vi "Main Page.vi"(8 "error in (no error)":errorcluster, 11 "Node Ptr":T3 format="%.0x") -> (0 "error out":errorcluster)   [LabVIEW 2026, in "Nominal Core Streaming System Explorer.lvlib"]
uses:
  Nominal Core Streaming System Explorer.lvlib
  <vilib>/NI VeriStand/Custom Device API/Custom Device Item Ref.ctl
  Shared/stream configuration mode.ctl
  <vilib>/NI VeriStand/Custom Device API/Get Item Property (U16).vi
  <vilib>/NI VeriStand/Custom Device API/Set Item Property (U16).vi
  <vilib>/NI VeriStand/Custom Device API/Custom Device API.lvlib
  Shared/Nominal Core Streaming Shared.lvlib
  <vilib>/NI VeriStand/Custom Device Tools/Custom Device Utility Library/Custom Device Utility Library.lvlib
panel:
  in  "tabs":T1(tab)
  in  "Name":string
  in  "Description":string
  out "Version":string
  in  "Async Timeout (ms)":u16
  in  "Channel buffer size":u32=512 min=10 max=1000000
  in  "Nominal Base URL":string="https://api.gov.nominal.io/api/"
  in  "visibility":bool
  in  "Nominal API Key":string
  in  "identifier selection":T2
  in  "Dataset RID":string
  in  "Asset RID":string
  in  "Dataset Name":string
  in  "Logged Channels":i32[](listbox)
  in  "Remove Channels":bool
  in  "Add Channels":bool
  # "This is a measure of responsiveness - low values will send batches to Nominal Core with more regularity, high values will be more efficient (up to a point). Consider setting to > 1 second of data with a max buffer size of 10k and a min size of 500 and tuning from there based on performance.\n\nBuffer size (samples) = \n    max ( 500, \n               min( 10000,\n                         10 sec * Loop rate (samples/sec)\n                       )\n             )\n\nMemory = Buffer size * [  ( # channels * 8 bytes/dbl ) + (1 time channel * 8 bytes) ]\n                = Buffer size * 8 * (# channels + 1) bytes"
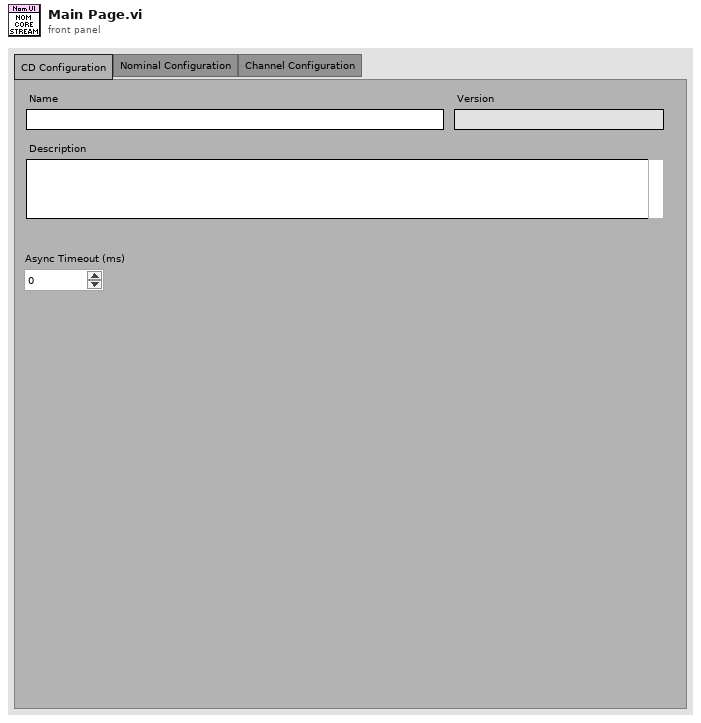
[diagram p1: front panel]
types:
  T1 = enum32{"CD Configuration", "Nominal Configuration", "Channel Configuration"}
  T2 = typedef "Nominal Core Streaming Shared.lvlib/stream configuration mode.ctl" = enum16{"Asset Identifier and Dataset Name", "Dataset Identifier"}
  T3 = typedef "Custom Device API.lvlib/Custom Device Item Ref.ctl" = u64
  T4 = typedef "Custom Device API.lvlib/Custom Device Item Info.ctl" = cluster{"Name":string, "Is Channel":bool, "GUID":string, "Is Waveform":bool}
  T5 = typedef "Custom Device API.lvlib/Custom Device Commands.ctl" = enum16{"Default", "Item renamed", "Shutdown", "Dynamic button pressed"}
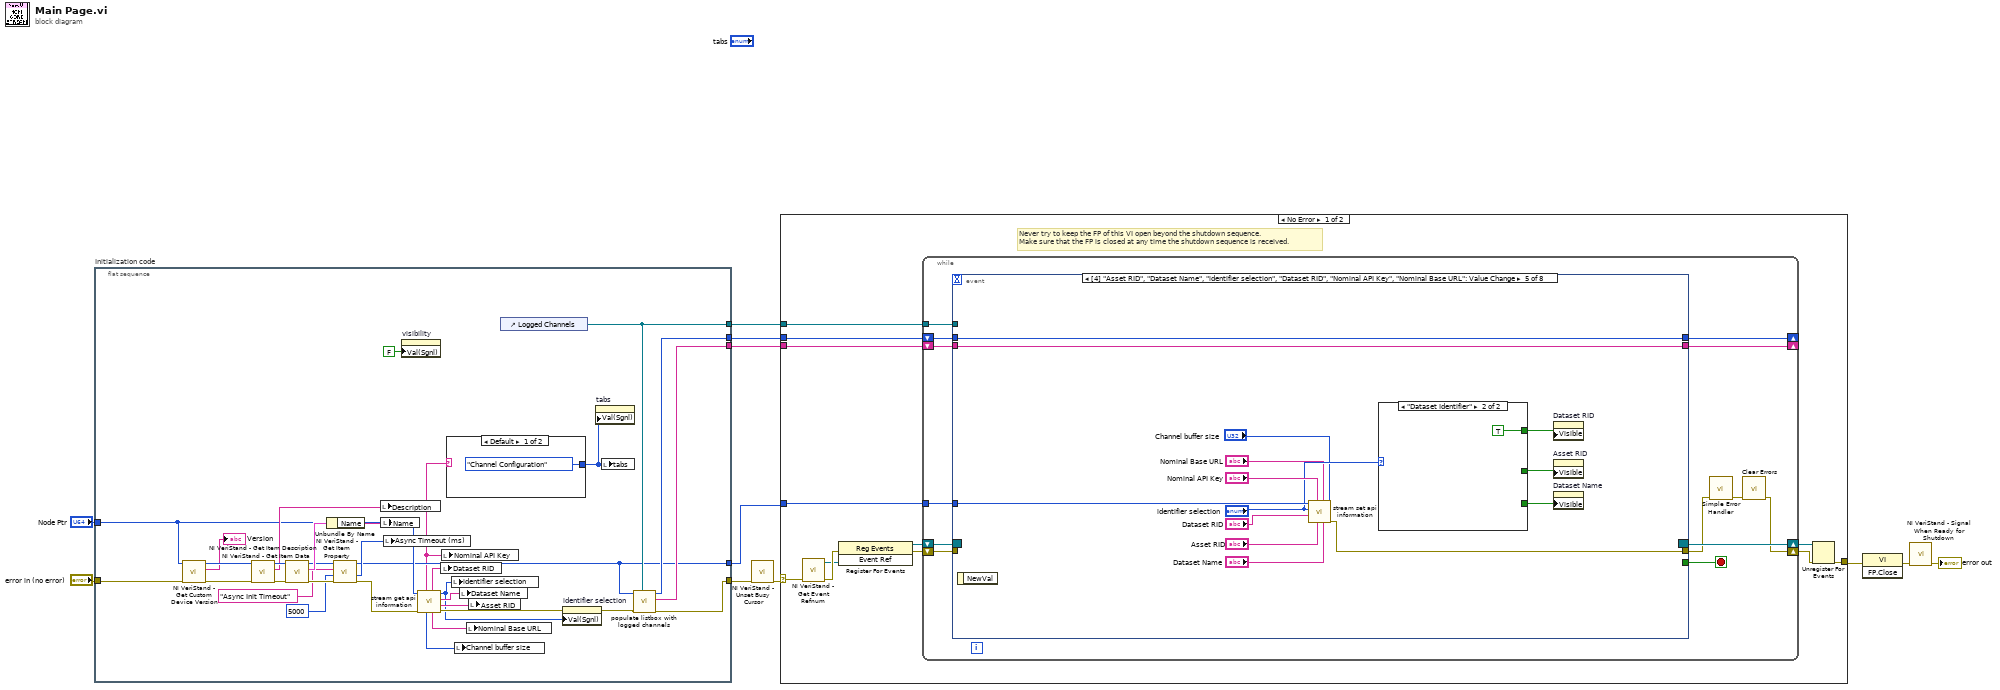
[diagram p0: block diagram]
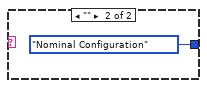
[diagram p2: hidden frame]
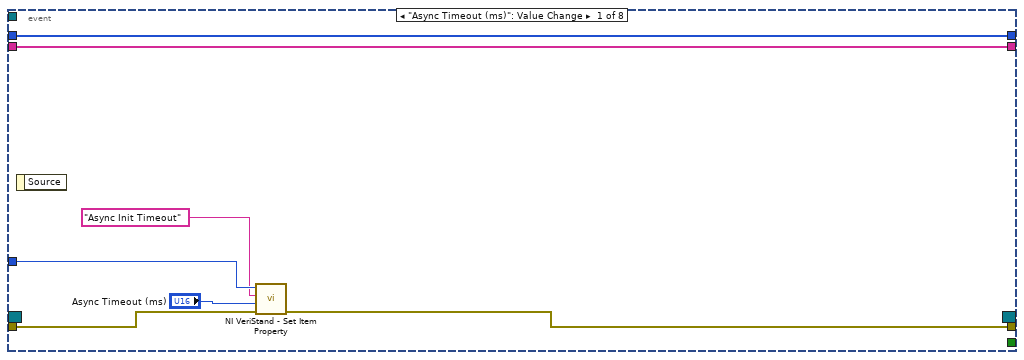
[diagram p3: hidden frame]
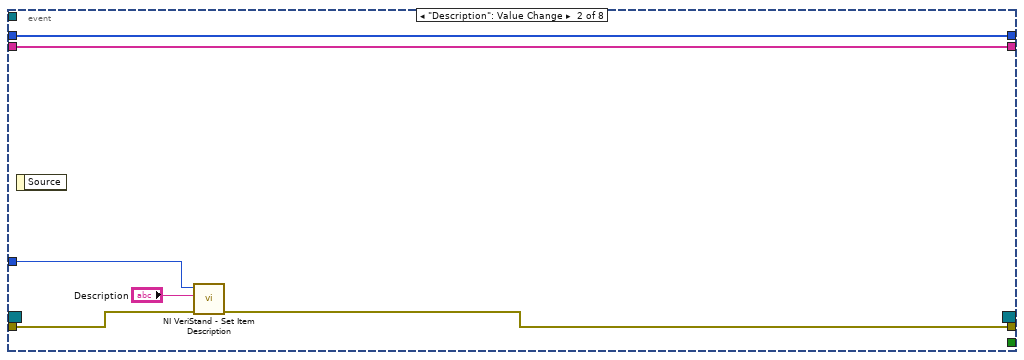
[diagram p4: hidden frame]
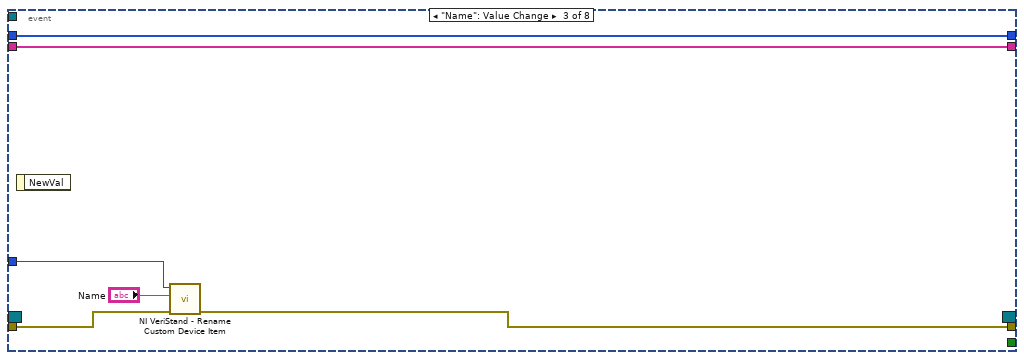
[diagram p5: hidden frame]
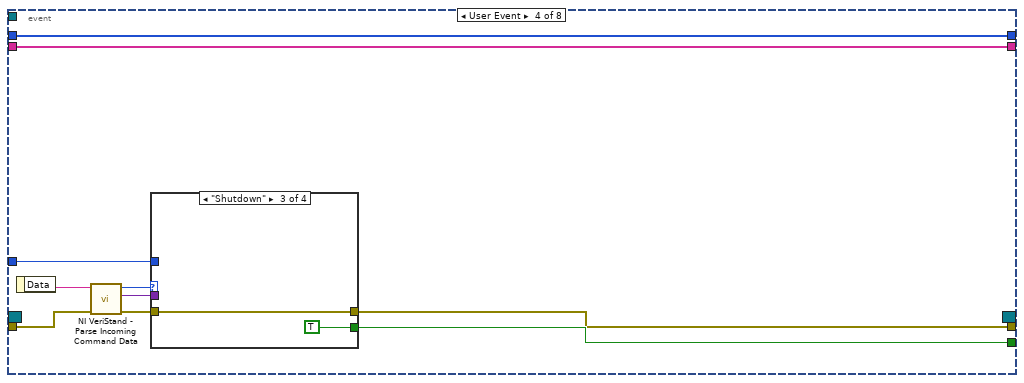
[diagram p6: hidden frame]
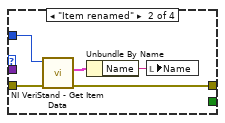
[diagram p8: hidden frame]
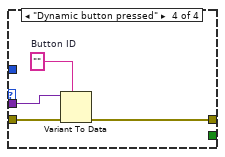
[diagram p9: hidden frame]
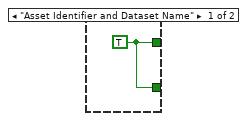
[diagram p10: hidden frame]
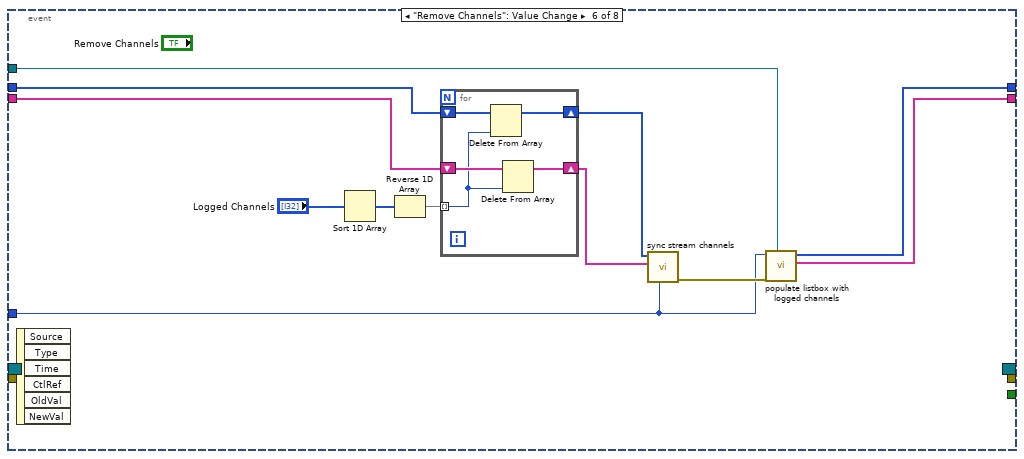
[diagram p11: hidden frame]
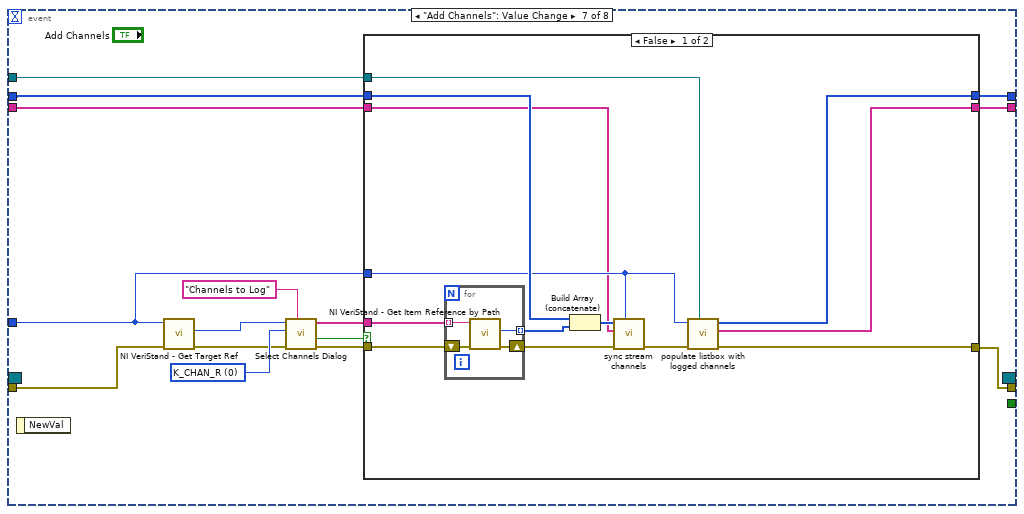
[diagram p12: hidden frame]
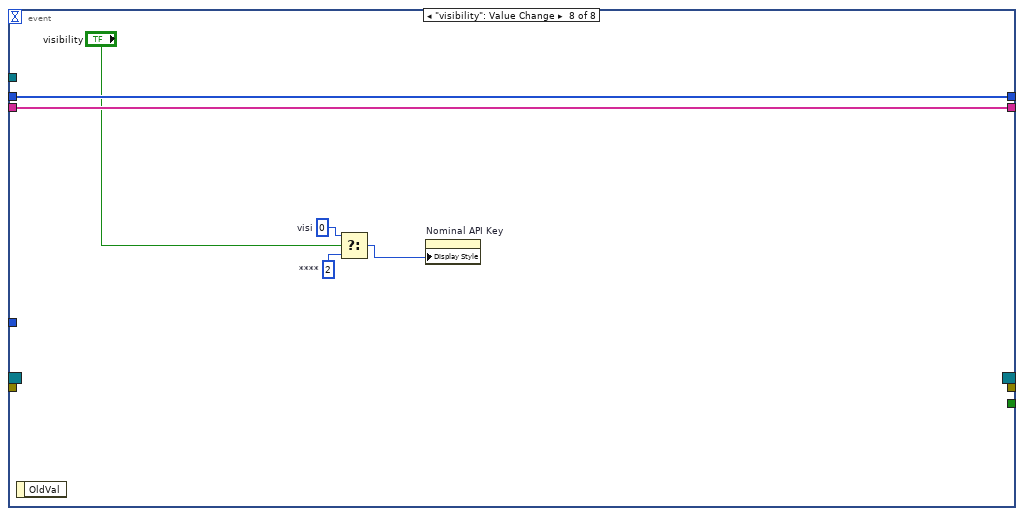
[diagram p14: hidden frame]
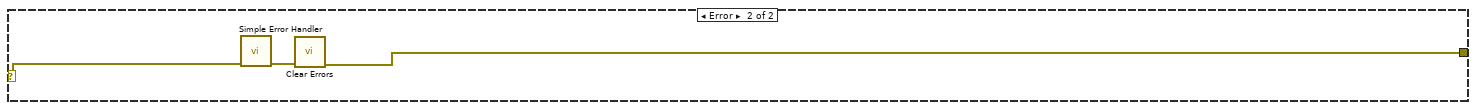
[diagram p15: hidden frame]
diagram:
  n1 = flat-sequence "Initialization code" {
    tunnel: "error in (no error)" -> [w35]
    tunnel: "Node Ptr" -> [w28]
    tunnel: [w24] -> w7
    tunnel: [w20] -> w4
    tunnel: [w21] -> w3
    tunnel: [w23] -> w2
    tunnel: [w22] -> w1
    frame #0 {
      n2 = call <vilib>:"NI VeriStand - Get Custom Device Version.vi"("error in (no error)"=w35, "Device Ref in"=w28) -> ("error out"=w40:errorcluster, "Value"=→"Version":string, "Device Ref out"=w39:T3)  [unwired: 7 in]
      n3 = call <vilib>:"NI VeriStand - Get Item Description.vi"("error in (no error)"=w40, "Item Ref in"=w39) -> ("error out"=w42:errorcluster, "Description"=w36:string, "Item Ref out"=w43:T3)  [unwired: 7 out]
      n4 = call <vilib>:"NI VeriStand - Get Item Data.vi"("error in (no error)"=w42, "Item Ref in"=w43) -> ("error out"=w34:errorcluster, "Item Info"=w41:T4, "Item Ref out"=w33:T3)  [unwired: 7 out]
      n5 = Unbundle By Name(w41) -> ("Name"=w37:string)
      n6 = call-poly <vilib>:"NI VeriStand - Get Item Property.vi"("error in (no error)"=w34, "Default Value"=u16 5000, "Property Name"="Async Init Timeout", "Item Ref in"=w33) -> ("error out"=w29:errorcluster, "Value"=w32:u16, "Item Ref out"=w20:T3)  [unwired: 4 in, 1 out]
      n7 = local write "Description"(w36) -> ()
      n8 = local write "Name"(w37) -> ()
      n9 = local write "Async Timeout (ms)"(w32) -> ()
      n10 = property on="visibility" class="Bool (strict)"("Val(Sgnl)"=FALSE ("Value (Signaling)")) -> ()  [unwired: 2 in, 2 out]
      n11 = call "stream get api information.vi"("error in"=w29, "CD in"=w28) -> ("error out"=w15:errorcluster, "asset ID"=w25:string, "dataset name"=w26:string, "ID selection"=w13:T2, "nominal base url"=w16:string, "dataset ID"=w27:string, "Channel buffer size"=w12:u32, "API key"=w19:string)  [unwired: 2 in]
      n12 = local write "Dataset RID"(w27) -> ()
      n13 = local write "Nominal API Key"(w19) -> ()
      n14 = case shown="Default" w19 {
        tunnel: [T1."Channel Configuration" ("tabs") T1."Nominal Configuration" ("tabs")] -> w17
        frame Default {
        }
        frame "" {
        }
      }
      n15 = local write "identifier selection"(w13) -> ()
      n16 = local write "Channel buffer size"(w12) -> ()
      n17 = local write "Dataset Name"(w26) -> ()
      n18 = local write "Nominal Base URL"(w16) -> ()
      n19 = local write "Asset RID"(w25) -> ()
      n20 = control-ref of="Logged Channels"() -> (w21:refnum<vi>)
      n21 = property on="identifier selection" class="Enum (strict)"(error in=w15, "Val(Sgnl)"=w13) -> (error out=w14:errorcluster)  [unwired: 1 in, 1 out]
      n22 = property on="tabs" class="TabCtl (strict)"("Val(Sgnl)"=w17) -> ()  [unwired: 2 in, 2 out]
      n23 = local write "tabs"(w17) -> ()
      n24 = call "populate listbox with logged channels.vi"("MulticolumnListbox in"=w21, "error in"=w14, "Item Ref in"=w20) -> ("error out"=w24:errorcluster, "logged channel shortnames"=w22:string[], "logged channel refs"=w23:T3[])  [unwired: 6 in]
    }
  }
  n25 = call <vilib>:"NI VeriStand - Unset Busy Cursor.vi"("error in (no error)"=w7) -> ("error out"=w6:errorcluster)  [unwired: 10 out]
  n26 = case shown="No Error" w6 {
    selector: w6 -> [w49 w188]
    tunnel: [w54 w186] -> w11
    tunnel: w4 -> [w50 _]
    tunnel: w3 -> [w48 _]
    tunnel: w2 -> [w47 _]
    tunnel: w1 -> [w46 _]
    frame No Error {
      # "Never try to keep the FP of this VI open beyond the shutdown sequence.\nMake sure that the FP is closed at any time the shutdown sequence is received."
      n27 = call <vilib>:"NI VeriStand - Get Event Refnum.vi"("error in (no error)"=w49) -> ("error out"=w57:errorcluster, "Event Ref"=w53:refnum<user-event>)  [unwired: 9 out]
      n28 = register-events(error in=w57, w53) -> (reference out=w51:refnum<event-registration>, error out=w52:errorcluster)  [unwired: 1 in]
      n29 = while {
        tunnel: w50 -> [w66]
        shift-right: [w63] -> w55
        shift-left: w52 -> [w69]
        shift-right: [w70] -> w56
        shift-left: w51 -> [w68]
        tunnel: w48 -> [w62]
        shift-right: [w59] -> _
        shift-left: w47 -> [w61]
        shift-right: [w58] -> _
        shift-left: w46 -> [w60]
        stop <- w67 stop-if-true
        n30 = event shown="[4] \"Asset RID\", \"Dataset Name\", \"identifier selection\", \"Dataset RID\", \"Nominal API Key\", \"Nominal Base URL\": Value Change" {
          selector: w68 -> [_ _ _ _ _ _ _ _]
          dyn-events: [_ _ _ _ _ _ _ _] -> w70
          timeout: _ -> [_ _ _ _ _ _ _ _]
          tunnel: w69 -> [w77 w82 w89 w99 _ _ w159 _]
          tunnel: [_ _ _ w95 _ _ _ _] -> w67
          tunnel: [w74 w81 w88 w94 w121 _ w147 _] -> w65
          tunnel: w66 -> [w76 w83 w87 w93 w125 w130 w146 _]
          tunnel: w62 -> [_ _ _ _ _ w134 w145 _]
          tunnel: w61 -> [w72 w79 w85 w91 w115 w133 w151 w185]
          tunnel: w60 -> [w71 w78 w84 w90 w114 w132 w150 w184]
          tunnel: [w72 w79 w85 w91 w115 w129 w152 w185] -> w59
          tunnel: [w71 w78 w84 w90 w114 w128 w149 w184] -> w58
          event "Async Timeout (ms)": Value Change {
            n31 = event-data() -> ()  [unwired: 2 out]
            n32 = call-poly <vilib>:"NI VeriStand - Set Item Property.vi"("error in (no error)"=w77, "Value"="Async Timeout (ms)", "Property Name"="Async Init Timeout", "Item Ref in"=w76) -> ("error out"=w74:errorcluster)  [unwired: 5 in, 2 out]
          }
          event "Description": Value Change {
            n33 = event-data() -> ()  [unwired: 2 out]
            n34 = call <vilib>:"NI VeriStand - Set Item Description.vi"("error in (no error)"=w82, "Description"="Description", "Item Ref in"=w83) -> ("error out"=w81:errorcluster)  [unwired: 8 out]
          }
          event "Name": Value Change {
            n35 = event-data() -> ()  [unwired: 2 out]
            n36 = call <vilib>:"NI VeriStand - Rename Custom Device Item.vi"("error in (no error)"=w89, "New Name"="Name", "Item Ref in"=w87) -> ("error out"=w88:errorcluster)  [unwired: 1 in, 7 out]
          }
          event User Event {
            n37 = event-data() -> ("Data"=w98:string)  [unwired: 1 out]
            n38 = call <vilib>:"NI VeriStand - Parse Incoming Command Data.vi"("error in (no error)"=w99, "Incoming data"=w98) -> ("error out"=w97:errorcluster, "Outgoing data"=w92:variant, "Action"=w96:T5)  [unwired: 7 out]
            n39 = case shown="\"Shutdown\"" w96 {
              tunnel: w97 -> [w100 w105 w106 w111]
              tunnel: [_ _ TRUE _] -> w95
              tunnel: [w100 w102 w106 w108] -> w94
              tunnel: w93 -> [_ w104 _ _]
              tunnel: w92 -> [_ _ _ w110]
              frame "Default", Default {
              }
              frame "Item renamed" {
                n40 = call <vilib>:"NI VeriStand - Get Item Data.vi"("error in (no error)"=w105, "Item Ref in"=w104) -> ("error out"=w102:errorcluster, "Item Info"=w103:T4)  [unwired: 8 out]
                n41 = Unbundle By Name(w103) -> ("Name"=w101:string)
                n42 = local write "Name"(w101) -> ()
              }
              frame "Shutdown" {
              }
              frame "Dynamic button pressed" {
                w109 = ""  # Button ID
                n43 = Variant To Data(error in=w111, type=w109, Variant=w110) -> (error out=w108:errorcluster)  [unwired: 1 out]
              }
            }
          }
          event "Asset RID", "Dataset Name", "Dataset RID", "Nominal API Key", "Nominal Base URL": Value Change {
            n44 = event-data() -> ()  [unwired: 2 out]
            n45 = call "stream set api information.vi"("Channel buffer size"="Channel buffer size", "dataset name"="Dataset Name", "Nominal Base URL"="Nominal Base URL", "asset ID"="Asset RID", "API key"="Nominal API Key", "dataset ID"="Dataset RID", "ID selection"="identifier selection", "CD in"=w125) -> ("error out"=w121:errorcluster)  [unwired: 3 in]
            n46 = case shown="\"Dataset Identifier\"" "identifier selection" {
              tunnel: [w126 _] -> w118
              tunnel: [w126 _] -> w117
              tunnel: [_ TRUE] -> w116
              frame "Asset Identifier and Dataset Name" {
                w126 = TRUE
              }
              frame "Dataset Identifier" {
              }
            }
            n47 = property on="Dataset RID" class="Str"("Visible"=w116) -> ()  [unwired: 2 in, 2 out]
            n48 = property on="Asset RID" class="Str"("Visible"=w118) -> ()  [unwired: 2 in, 2 out]
            n49 = property on="Dataset Name" class="Str"("Visible"=w117) -> ()  [unwired: 2 in, 2 out]
          }
          event "Remove Channels": Value Change {
            n50 = event-data() -> ()  [unwired: 7 out]
            n51 = Sort 1D Array(array="Logged Channels") -> (sorted array=w137:i32[])
            n52 = Reverse 1D Array(array=w137) -> (reversed array=w138:i32[])
            n53 = for {
              tunnel: w138 -> [w140] mode=indexing
              shift-right: [w143] -> w131
              shift-left: w133 -> [w144]
              shift-right: [w141] -> w139
              shift-left: w132 -> [w142]
              n54 = Delete From Array(array=w144, index=w140) -> (array with subset deleted=w143:T3[])  [unwired: 1 in, 1 out]
              n55 = Delete From Array(array=w142, index=w140) -> (array with subset deleted=w141:string[])  [unwired: 1 in, 1 out]
            }
            n56 = call "sync stream channels.vi"("stream"=w130, "names"=w139, "channels"=w131) -> ("error out"=w136:errorcluster)  [unwired: 6 in, 2 out]
            n57 = call "populate listbox with logged channels.vi"("MulticolumnListbox in"=w134, "error in"=w136, "Item Ref in"=w130) -> ("logged channel shortnames"=w128:string[], "logged channel refs"=w129:T3[])  [unwired: 6 in, 1 out]
          }
          event "Add Channels": Value Change {
            w158 = u8 0 items=["K_CHAN_R", "K_CHAN_W", "K_CHAN_RW", "K_CHAN_VOLT", "K_CHAN_FAULT", "K_ALL", "K_CUSTOM"] ("Filter")
            n58 = event-data() -> ()  [unwired: 2 out]
            n59 = call <vilib>:"NI VeriStand - Get Target Ref.vi"("error in"=w159, "Item Ref in"=w146) -> ("error out"=w156:errorcluster, "Target Ref"=w155:T3)  [unwired: 6 in, 2 out]
            n60 = call "Select Channels Dialog.vi"("Tree header"="Channels to Log", "error in (no error)"=w156, "Filter"=w158, "Start Item Ref"=w155) -> ("error out"=w153:errorcluster, "Canceled"=w154:bool, "Channel paths"=w148:string[])  [unwired: 5 in]
            n61 = case shown="False" w154 {
              tunnel: w153 -> [w168 w177]
              tunnel: [w163 w179] -> w152
              tunnel: w151 -> [w165 w179]
              tunnel: w150 -> [w160 w178]
              tunnel: [w162 w178] -> w149
              tunnel: w148 -> [w167 _]
              tunnel: [w166 w177] -> w147
              tunnel: w146 -> [w161 _]
              tunnel: w145 -> [w164 _]
              frame False {
                n62 = for {
                  shift-right: [w175] -> w169
                  shift-left: w168 -> [w176]
                  tunnel: w167 -> [w174] mode=indexing
                  tunnel: [w173] -> w170 mode=indexing
                  n63 = call <vilib>:"NI VeriStand - Get Item Reference by Path.vi"("error in (no error)"=w176, "Item Path in"=w174) -> ("error out"=w175:errorcluster, "Item Ref"=w173:T3)  [unwired: 6 in, 2 out]
                }
                n64 = Build Array (concatenate)(w165, w170) -> (w171:T3[])
                n65 = call "sync stream channels.vi"("stream"=w161, "error in"=w169, "names"=w160, "channels"=w171) -> ("error out"=w172:errorcluster)  [unwired: 5 in, 2 out]
                n66 = call "populate listbox with logged channels.vi"("MulticolumnListbox in"=w164, "error in"=w172, "Item Ref in"=w161) -> ("error out"=w166:errorcluster, "logged channel shortnames"=w162:string[], "logged channel refs"=w163:T3[])  [unwired: 6 in]
              }
              frame True {
              }
            }
          }
          event "visibility": Value Change {
            w183 = u32 2  # ****
            w180 = u32 0  # visi
            n67 = event-data() -> ()  [unwired: 2 out]
            n68 = Select(t=w180, s="visibility", f=w183) -> (s? t:f=w182:u32)
            n69 = property on="Nominal API Key" class="Str"("Display Style"=w182) -> ()  [unwired: 2 in, 2 out]
          }
        }
        n70 = call <vilib>:"Simple Error Handler.vi"("error in (no error)"=w65) -> ("error out"=w64:errorcluster)  [unwired: 1 in, 7 out]
        n71 = call <vilib>:"Clear Errors.vi"("error in (no error)"=w64) -> ("error out"=w63:errorcluster)  [unwired: 1 in, 5 out]
      }
      n72 = Unregister For Events(event registration refnum=w56, error in=w55) -> (error out=w54:errorcluster)
    }
    frame Error {
      n73 = call <vilib>:"Simple Error Handler.vi"("error in (no error)"=w188) -> ("error out"=w187:errorcluster)  [unwired: 1 in, 7 out]
      n74 = call <vilib>:"Clear Errors.vi"("error in (no error)"=w187) -> ("error out"=w186:errorcluster)  [unwired: 1 in, 5 out]
    }
  }
  n75 = invoke class="VI" method="FP.Close"(error in=w11) -> (error out=w10:errorcluster)  [unwired: 2 in, 2 out]
  n76 = call <vilib>:"NI VeriStand - Signal When Ready for Shutdown.vi"("error in (no error)"=w10) -> ("error out"=→"error out":errorcluster)  [unwired: 10 out]
